vi "Downhill Simplex nD Value.vi"(1 "X":dbl[](array[numeric]) format="%.2f") -> (0 "f(X)":dbl format="%.2f")   [LabVIEW 2010, in "NI_Gmath.lvlib"]
uses:
  NI_Gmath.lvlib
  Downhill Simplex nD Global.vi
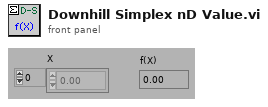
[diagram p1: front panel]
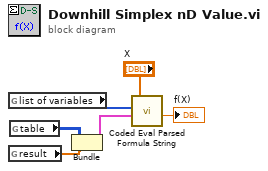
[diagram p0: block diagram]
diagram:
  n1 = global read "Downhill Simplex nD Global.vi" "list of variables"() -> (w1:i32[])
  n2 = global read "Downhill Simplex nD Global.vi" "result"() -> (w4:dbl[])
  n3 = global read "Downhill Simplex nD Global.vi" "table"() -> (w5:i32[][])
  n4 = Bundle("table"=w5, "result"=w4) -> (w3:cluster{"table":i32[][], "result":dbl[]})  [unwired: 1 in]
  n5 = call "Coded Eval Parsed Formula String.vi"("Parsed Formula"=w3, "Variables"=w1, "X Values"="X") -> ("y value"=→"f(X)":dbl)  [unwired: 1 in, 1 out]
